vi "Visual Cue Builder.vi"(10 "fixed array":i32[](array[numeric]), 11 "Loop Counter":i32) -> (2 "Trigger Point":bool, 3 "Array":i32[][](array[numeric]))   [LabVIEW 2019, in "CML UI.lvlib"]
uses:
  CML UI.lvlib
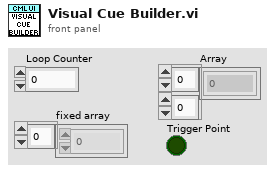
[diagram p1: front panel]
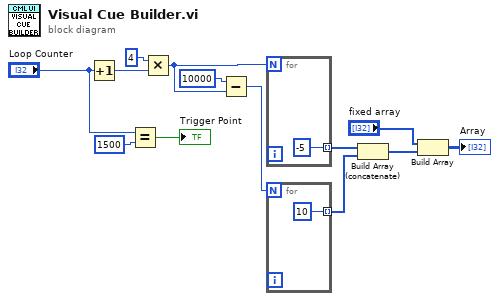
[diagram p0: block diagram]
diagram:
  n1 = Increment(x="Loop Counter") -> (x+1=w8:i32)
  n2 = Equal?(x="Loop Counter", y=1500) -> (x = y?=→"Trigger Point":bool)
  n3 = Multiply(x=4, y=w8) -> (x*y=w10:i32)
  n4 = Subtract(x=10000, y=w10) -> (x-y=w9:i32)
  n5 = for {
    N: w10 -> [_]
    tunnel: [-5] -> w5 mode=indexing
  }
  n6 = for {
    N: w9 -> [_]
    tunnel: [10] -> w4 mode=indexing
  }
  n7 = Build Array (concatenate)(w5, w4) -> (w6:i32[])
  n8 = Build Array("fixed array", w6) -> (→"Array":i32[][])
